vi "tree demo.vi"() -> ()   [LabVIEW 2010]
panel:
  out "Tree 2":string(tree)
  in  "stop":bool
  out "Active Item Properties:Active Item Tag":string
  in  "Tree":string(tree)
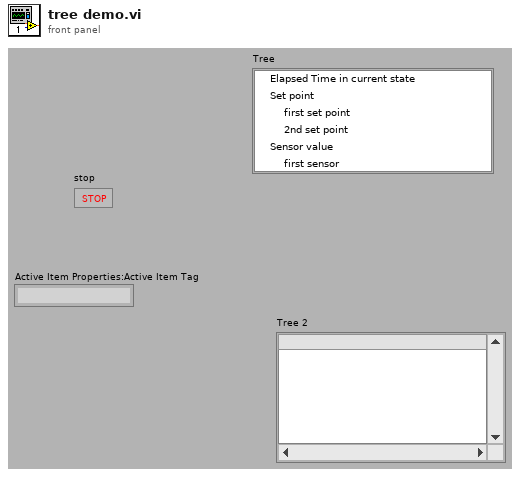
[diagram p1: front panel]
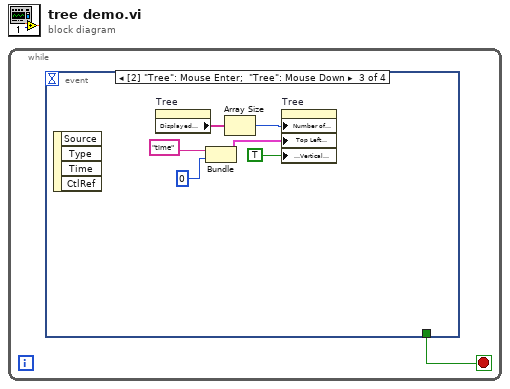
[diagram p0: block diagram]
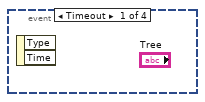
[diagram p2: hidden frame]
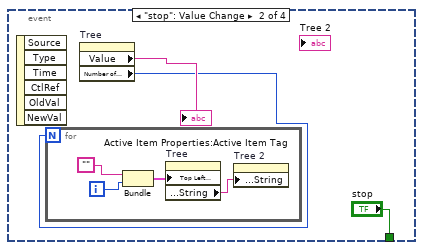
[diagram p3: hidden frame]
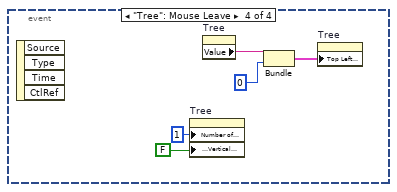
[diagram p4: hidden frame]
diagram:
  n1 = while {
    stop <- w1 stop-if-true
    n2 = event shown="[2] \"Tree\": Mouse Enter;  \"Tree\": Mouse Down" {
      selector: _ -> [_ _ _ _]
      dyn-events: _ -> [_ _ _ _]
      timeout: _ -> [_ _ _ _]
      tunnel: [_ "stop" _ _] -> w1
      event Timeout {
        n3 = event-data() -> ()  [unwired: 1 in, 2 out]
      }
      event "stop": Value Change {
        n4 = event-data() -> ()  [unwired: 1 in, 6 out]
        n5 = property on="Tree" class="Tree (strict)"() -> ("Value"=→"Active Item Properties:Active Item Tag":string, "Number of Rows"=w2:u32)  [unwired: 2 in, 2 out]
        n6 = for {
          N: w2 -> [_]
          i -> [w7]
          n7 = Bundle("", w7) -> (w6:cluster{string, i32})  [unwired: 1 in]
          n8 = property on="Tree" class="Tree (strict)"("Top Left Visible Cell"=w6) -> ("Active Cell:String"=w8:string)  [unwired: 2 in, 2 out]
          n9 = property on="Tree 2" class="Tree (strict)"("Active Cell:String"=w8) -> ()  [unwired: 2 in, 2 out]
        }
      }
      event "Tree": Mouse Enter; "Tree": Mouse Down {
        n10 = event-data() -> ()  [unwired: 1 in, 4 out]
        n11 = property on="Tree" class="Tree (strict)"() -> ("Displayed Items"=w14:string[])  [unwired: 2 in, 2 out]
        n12 = Bundle("Tree"="time", "Num Columns"=u32 0) -> (w10:cluster{"Tree":string, "Num Columns":u32})  [unwired: 1 in]
        n13 = Array Size(array=w14) -> (size(s)=w13:i32)
        n14 = property on="Tree" class="Tree (strict)"("Number of Rows"=w13, "Top Left Visible Cell"=w10, "Visible Items:Vertical Scrollbar Visible"=TRUE) -> ()  [unwired: 2 in, 2 out]
      }
      event "Tree": Mouse Leave {
        n15 = event-data() -> ()  [unwired: 1 in, 4 out]
        n16 = property on="Tree" class="Tree (strict)"("Number of Rows"=u32 1 ("Num Columns"), "Visible Items:Vertical Scrollbar Visible"=FALSE) -> ()  [unwired: 2 in, 2 out]
        n17 = property on="Tree" class="Tree (strict)"() -> ("Value"=w18:string)  [unwired: 2 in, 2 out]
        n18 = Bundle("Value"=w18, "Num Columns"=u32 0) -> (w17:cluster{"Value":string, "Num Columns":u32})  [unwired: 1 in]
        n19 = property on="Tree" class="Tree (strict)"("Top Left Visible Cell"=w17) -> ()  [unwired: 2 in, 2 out]
      }
    }
  }
